vi "ep_Split Spectra Symetrical Components.vi"(0 "complex spectra (5Hz step)":T3(array[cluster]), 7 "line voltage? (F)":bool, 11 "error in (no error)":errorcluster) -> (4 "spectra symetrical components":T1, 15 "error out":errorcluster)   [LabVIEW 2014, in "NI_EP_Power Quality.lvlib"]
uses:
  <vilib>/addons/Electrical Power/PQ/NI_EP_Power Quality.lvlib
  <vilib>/addons/Electrical Power/PQ/Common/Controls/ep_AI Data Channel.ctl
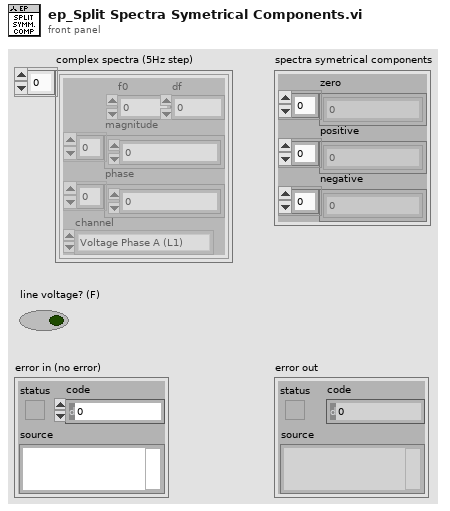
[diagram p1: front panel]
types:
  T1 = cluster{"zero":cdb[], "positive":cdb[], "negative":cdb[]}
  T2 = typedef "NI_EP_Power Quality.lvlib/ep_AI Data Channel.ctl" = enum16{"Voltage Phase A (L1)", "Voltage Phase B (L2)", "Voltage Phase C (L3)", "Voltage Phase N (Neutral)", "Current Phase A (L1)", "Current Phase B (L2)", "Current Phase C (L3)", "Current Phase N (Neutral)"}
  T3 = cluster{"f0":dbl, "df":dbl, "magnitude":dbl[], "phase":dbl[], "channel":T2}[]
  T4 = cluster{"f0":dbl, "df":dbl, "magnitude":dbl[], "phase":dbl[], "channel":T2}
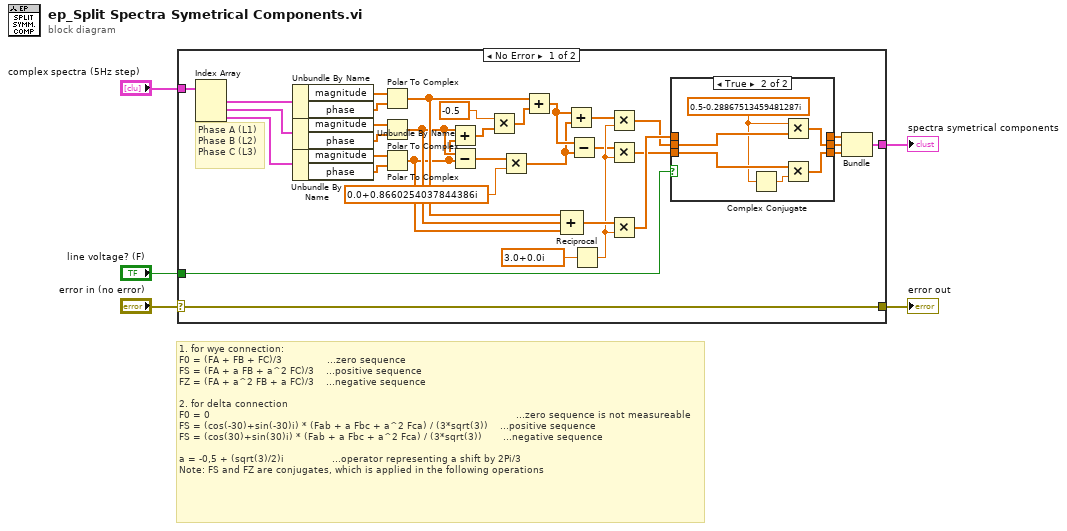
[diagram p0: block diagram]
diagram:
  # "1. for wye connection:\nF0 = (FA + FB + FC)/3               ...zero sequence\nFS = (FA + a FB + a^2 FC)/3    ...positive sequence\nFZ = (FA + a^2 FB + a FC)/3    ...negative sequence\n\n2. for delta connection\nF0 = 0                                                                                                      ...zero sequence is not measureable\nFS = (cos(-30)+sin(-30)i) * (Fab + a Fbc + a^2 Fca) / (3*sqrt(3))    ...positive sequence\nFS = (cos(30)+sin(30)i) * (Fab + a Fbc + a^2 Fca) / (3*sqrt(3))       ...negative sequence\n\na = -0,5 + (sqrt(3)/2)i                ...operator representing a shift by 2Pi/3\nNote: FS and FZ are conjugates, which is applied in the following operations"
  n1 = case shown="No Error" "error in (no error)" {
    selector: "error in (no error)" -> [w13 w49]
    tunnel: "complex spectra (5Hz step)" -> [w34 _]
    tunnel: [w14 _] -> w4
    tunnel: [w13 w49] -> w2
    tunnel: "line voltage? (F)" -> [w6 _]
    frame No Error {
      # "Phase A (L1)\nPhase B (L2)\nPhase C (L3)"
      n2 = Index Array(array=w34) -> (element #1=w38:T4, element #2=w37:T4, element #3=w36:T4)  [unwired: 3 in]
      n3 = Unbundle By Name(w38) -> ("magnitude"=w32:dbl[], "phase"=w31:dbl[])
      n4 = Unbundle By Name(w37) -> ("magnitude"=w29:dbl[], "phase"=w30:dbl[])
      n5 = Unbundle By Name(w36) -> ("magnitude"=w27:dbl[], "phase"=w28:dbl[])
      n6 = Polar To Complex(1:w31, 2:w32) -> (0:w17:cdb[])
      n7 = Polar To Complex(1:w30, 2:w29) -> (0:w16:cdb[])
      n8 = Polar To Complex(1:w28, 2:w27) -> (0:w15:cdb[])
      n9 = Add(x=w16, y=w15) -> (x+y=w26:cdb[])
      n10 = Subtract(x=w16, y=w15) -> (x-y=w23:cdb[])
      n11 = Multiply(x=-0.5 ("y"), y=w26) -> (x*y=w24:cdb[])
      n12 = Multiply(x=w23, y=cdb 0.0+0.8660254037844386i) -> (x*y=w20:cdb[])
      n13 = Add(x=w17, y=w24) -> (x+y=w21:cdb[])
      n14 = Compound Arithmetic op=ADD(w17, w16, w15) -> (w35:cdb[])
      n15 = Add(x=w21, y=w20) -> (x+y=w19:cdb[])
      n16 = Subtract(x=w21, y=w20) -> (x-y=w18:cdb[])
      n17 = Reciprocal(x=cdb 3.0+0.0i ("y")) -> (1/x=w33:cdb)
      n18 = Multiply(x=w19, y=w33) -> (x*y=w10:cdb[])
      n19 = Multiply(x=w18, y=w33) -> (x*y=w7:cdb[])
      n20 = Multiply(x=w35, y=w33) -> (x*y=w12:cdb[])
      n21 = case shown="True" w6 {
        tunnel: w12 -> [w42 _]
        tunnel: [w42 _] -> w11
        tunnel: w10 -> [w41 w48]
        tunnel: [w41 w47] -> w9
        tunnel: [w40 w45] -> w8
        tunnel: w7 -> [w40 w46]
        frame False {
        }
        frame True {
          w43 = cdb 0.5-0.28867513459481287i
          n22 = Complex Conjugate(1:w43) -> (0:w44:cdb)
          n23 = Multiply(x=w43, y=w48) -> (x*y=w47:cdb[])
          n24 = Multiply(x=w46, y=w44) -> (x*y=w45:cdb[])
        }
      }
      n25 = Bundle(w11, w9, w8) -> (w14:cluster{cdb[], cdb[], cdb[]})  [unwired: 1 in]
    }
    frame Error {
    }
  }
  "spectra symetrical components" <- w4
  "error out" <- w2
